vi "SetupSweepAndGetPeak.vi"(6 "Route Names":string[](array[string]), 7 "Cal?":bool=TRUE, 8 "error in (no error)":errorcluster, 9 "Span(Hz)":dbl=26500000000.0, 10 "Center Frequency(Hz)":dbl=13250000000.0, 11 "PwrMtr_U2k in":refnum<class "PwrMtr_U2k.lvclass">) -> (0 "error out":errorcluster, 1 "FDelta(hz)":dbl, 2 "Calibrated Amplitude (dBm)":dbl, 3 "PwrMtr_U2k out":refnum<class "PwrMtr_U2k.lvclass">)   [LabVIEW 2014, in "PwrMtr_U2k.lvclass"]
uses:
  PwrMtr_U2k.lvclass
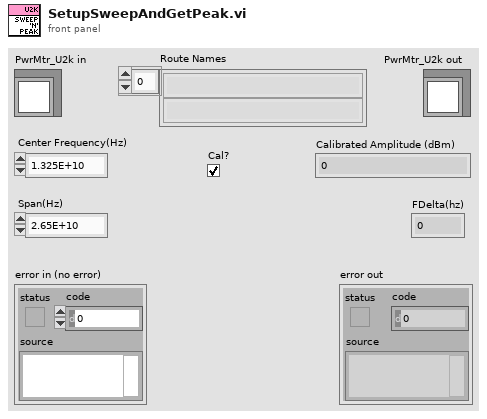
[diagram p1: front panel]
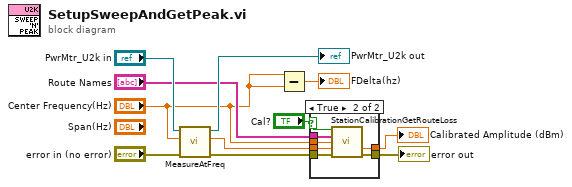
[diagram p0: block diagram]
diagram:
  n1 = call-dynamic "MeasureAtFreq.vi"("error in (no error)"="error in (no error)", "Frequency (Hz)"="Center Frequency(Hz)", "PwrMtr_U2k in"="PwrMtr_U2k in") -> ("error out"=w6:errorcluster, "Power (dBm)"=w7:dbl, "PwrMtr_U2k out"=→"PwrMtr_U2k out":refnum<class "PwrMtr_U2k.lvclass">)  [unwired: 6 in]
  n2 = Subtract(x="Center Frequency(Hz)", y="Center Frequency(Hz)") -> (x-y=→"FDelta(hz)":dbl)
  n3 = case shown="True" "Cal?" {
    selector: "Cal?" -> [_ w14]
    tunnel: [w13 w20] -> w9
    tunnel: "Route Names" -> [_ w19]
    tunnel: "Center Frequency(Hz)" -> [_ w18]
    tunnel: w7 -> [w13 w17]
    tunnel: w6 -> [w12 w16]
    tunnel: [w12 w15] -> w4
    frame False {
    }
    frame True {
      n4 = call "StationCalibrationGetRouteLoss.vi"("Calibration Enabled"=w14, "Route Names"=w19, "Frequency"=w18, "Power Level"=w17, "error in (no error)"=w16) -> ("Adjusted Power Level"=w20:dbl, "error out"=w15:errorcluster)  [unwired: 7 in, 2 out]
    }
  }
  "error out" <- w4
  "Calibrated Amplitude (dBm)" <- w9
